vi "UTILITY Release Semaphore.vi"(8 "error in (no error)":errorcluster, 9 "Debug":bool, 11 "Refnum in":T1) -> (0 "error out":errorcluster)   [LabVIEW 2019]
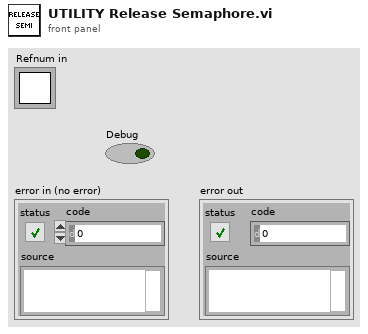
[diagram p1: front panel]
types:
  T1 = typedef "Semaphore RefNum" = refnum<k1>
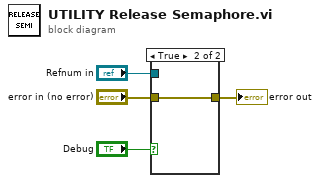
[diagram p0: block diagram]
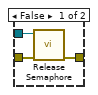
[diagram p2: hidden frame]
diagram:
  n1 = case shown="True" "Debug" {
    tunnel: "error in (no error)" -> [w7 w8]
    tunnel: [w6 w8] -> w3
    tunnel: "Refnum in" -> [w5 _]
    frame False {
      n2 = call <vilib>:"Release Semaphore.vi"("error in (no error)"=w7, "semaphore"=w5) -> ("error out"=w6:errorcluster)  [unwired: 4 in, 1 out]
    }
    frame True {
    }
  }
  "error out" <- w3
